vi "Spartan HTTP Load Global Resource Configuration.vi"(8 "error in (no error)":errorcluster) -> (0 "error out":errorcluster)   [LabVIEW 2011]
uses:
  ITK EXT/http/http0.llb/HTTP LVHTTP Global.vi
  ITK EXT/http/config.llb/HTTP SRM.vi
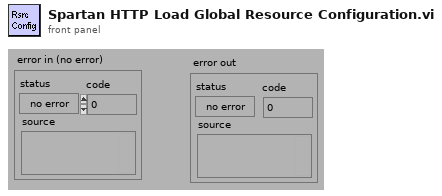
[diagram p1: front panel]
types:
  T1 = typedef "Keyed Array.ctl" = cluster{"keys":string[], "values":string[]}
  T2 = enum32{"noop", "DocumentRoot", "UserDir", "AccessFileName", "DefaultType", "DefaultIcon", "DirectoryIndex", "ReadmeName", "HeaderName", "ErrorDocument", "FancyIndexing", "IndexIgnore", "IndexOption", "Redirect", "Alias", "ScriptAlias", "AddType", "AddEncoding", "AddDescription", "AddIcon", "AddIconByType", "AddIconByEncoding"}
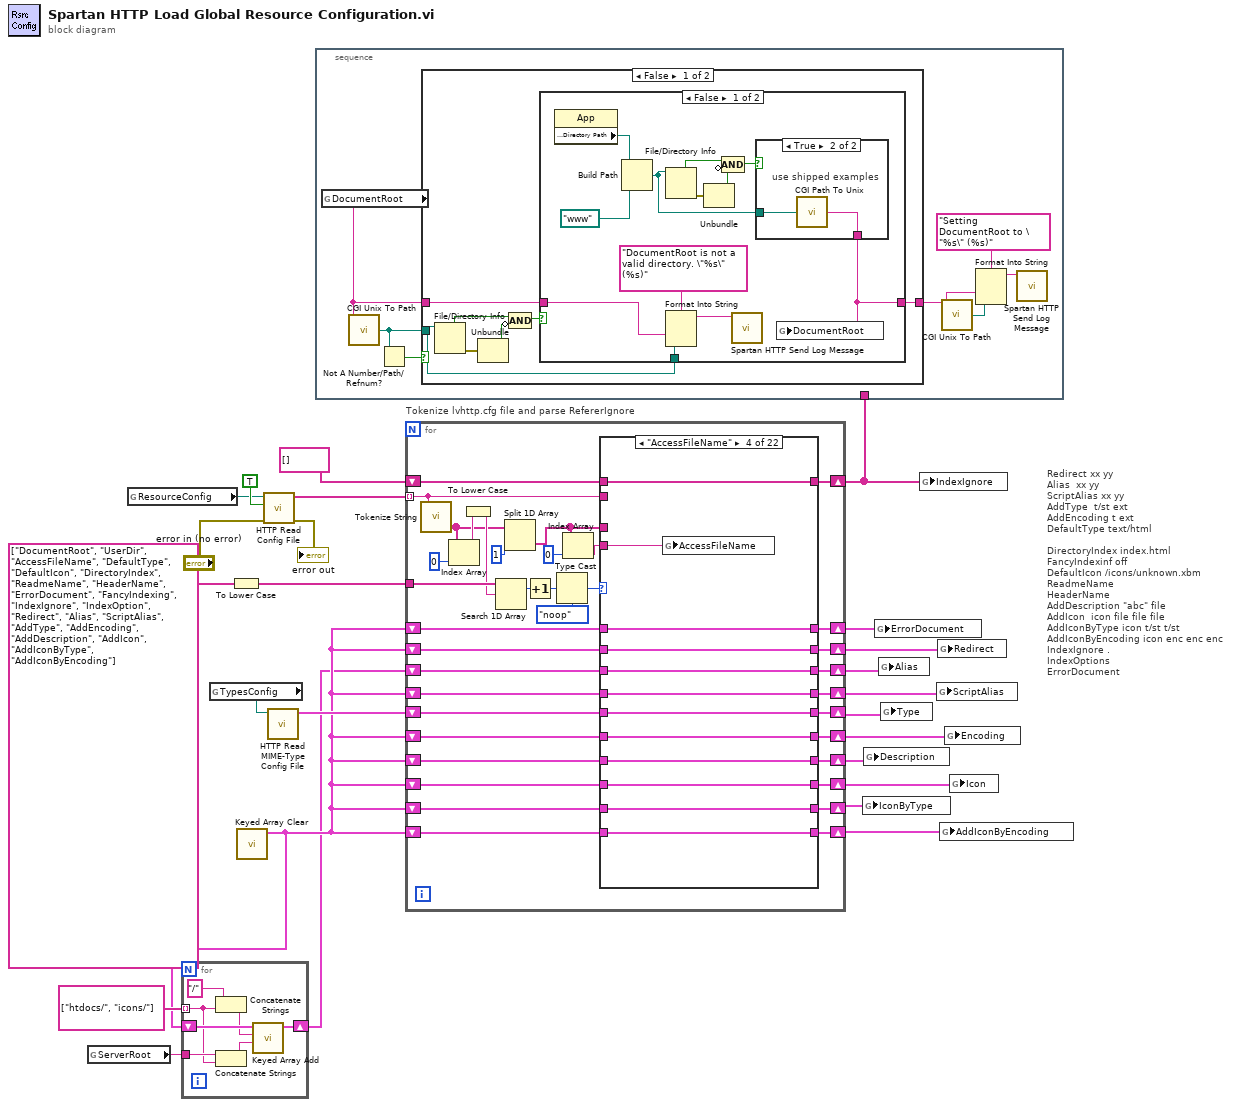
[diagram p0: block diagram]
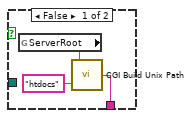
[diagram p2: hidden frame]
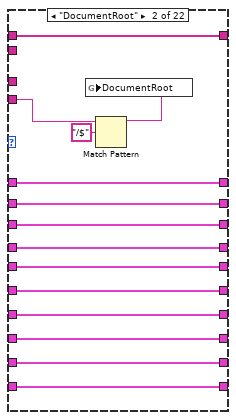
[diagram p6: hidden frame]
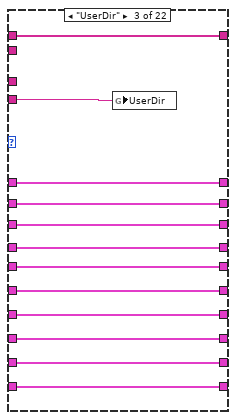
[diagram p7: hidden frame]
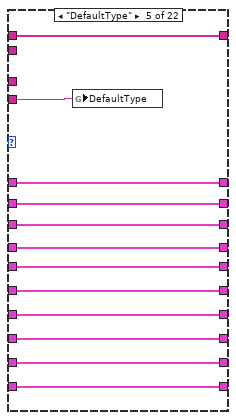
[diagram p8: hidden frame]
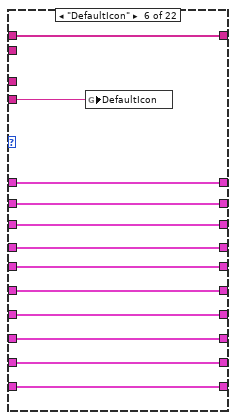
[diagram p9: hidden frame]
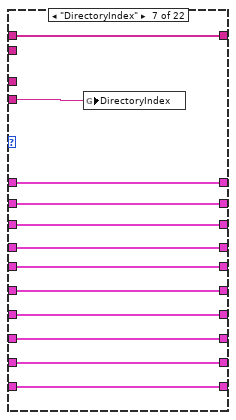
[diagram p10: hidden frame]
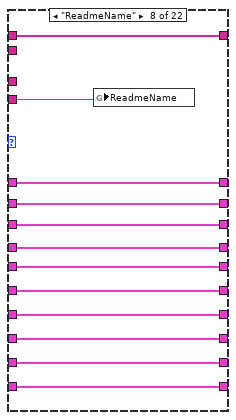
[diagram p11: hidden frame]
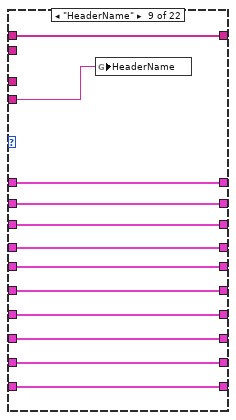
[diagram p12: hidden frame]
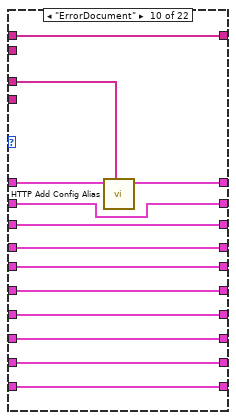
[diagram p13: hidden frame]
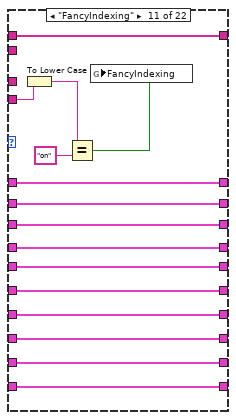
[diagram p14: hidden frame]
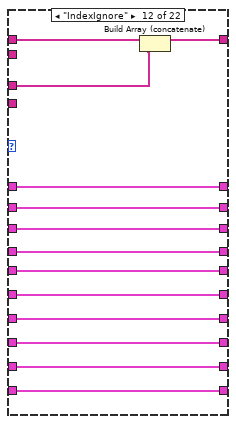
[diagram p15: hidden frame]
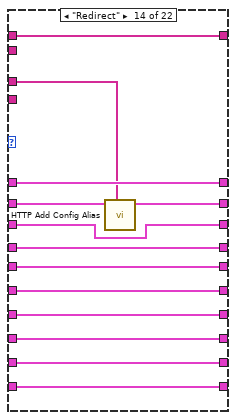
[diagram p17: hidden frame]
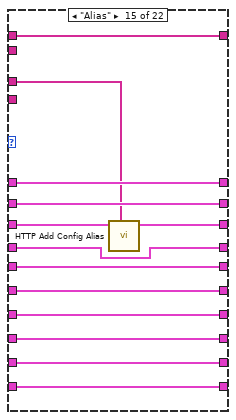
[diagram p18: hidden frame]
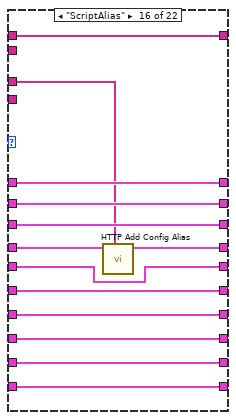
[diagram p19: hidden frame]
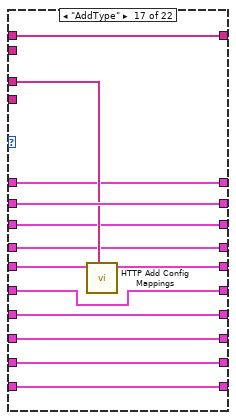
[diagram p20: hidden frame]
diagram:
  # "Redirect\txx yy\nAlias\t\txx yy\nScriptAlias\txx yy\nAddType\t\tt/st ext\nAddEncoding\tt ext\nDefaultType\ttext/html\n\nDirectoryIndex\tindex.html\nFancyIndexinf\toff\nDefaultIcon\t/icons/unknown.xbm\nReadmeName\nHeaderName\nAddDescription\t\"abc\" file\nAddIcon\t\ticon file file file\nAddIconByType\ticon t/st t/st\nAddIconByEncoding\ticon enc enc enc\nIndexIgnore\t.\nIndexOptions\nErrorDocument"
  n1 = global read "HTTP LVHTTP Global.vi" "ServerRoot"() -> (w14:string)
  n2 = global read "HTTP LVHTTP Global.vi" "ResourceConfig"() -> (w17:path)
  n3 = global read "HTTP LVHTTP Global.vi" "TypesConfig"() -> (w25:path)
  n4 = To Lower Case(string=string[] ["DocumentRoot", "UserDir", "AccessFileName", "DefaultType", "DefaultIcon", "DirectoryIndex", "ReadmeName", "HeaderName", "ErrorDocument", "FancyIndexing", "IndexIgnore", "IndexOption", "Redirect", "Alias", "ScriptAlias", "AddType", "AddEncoding", "AddDescription", "AddIcon", "AddIconByType", "AddIconByEncoding"] ("token array")) -> (all lower case string=w16:string[])
  n5 = call "Keyed Array Clear.vi"() -> ("array out"=w13:T1)  [unwired: 1 in, 6 out]
  n6 = for {
    shift-right: [w31] -> w12
    shift-left: w13 -> [w32]
    tunnel: string[] ["htdocs/", "icons/"] -> [w27] mode=indexing
    tunnel: w14 -> [w28]
    n7 = Concatenate Strings("/", w27) -> (w29:string)
    n8 = Concatenate Strings(w28, w27) -> (w26:string)
    n9 = call "Keyed Array Add.vi"("value"=w26, "key"=w29, "array in"=w32) -> ("array out"=w31:T1)  [unwired: 1 in, 3 out]
  }
  n10 = call "HTTP Read Config File.vi"("error in (no error)"="error in (no error)", "skip blank lines (F)"=TRUE, "config file path"=w17) -> ("error out"=→"error out":errorcluster, "lines"=w22:string[])  [unwired: 7 out]
  n11 = call "HTTP Read MIME-Type Config File.vi"("mime.types config file path"=w25) -> ("mime mapping"=w18:T1)  [unwired: 1 in, 9 out]
  n12 = for "Tokenize lvhttp.cfg file and parse RefererIgnore" {
    shift-right: [w47] -> w9
    shift-left: w13 -> [w68]
    tunnel: w22 -> [w40] mode=indexing
    shift-right: [w66] -> w11
    shift-left: string[] [] -> [w67]
    tunnel: w16 -> [w65]
    shift-right: [w60] -> w8
    shift-left: w12 -> [w61]
    shift-right: [w59] -> w7
    shift-left: w13 -> [w58]
    shift-right: [w56] -> w6
    shift-left: w18 -> [w57]
    shift-right: [w54] -> w5
    shift-left: w13 -> [w55]
    shift-right: [w53] -> w4
    shift-left: w13 -> [w46]
    shift-right: [w52] -> w3
    shift-left: w13 -> [w51]
    shift-right: [w50] -> w2
    shift-left: w13 -> [w49]
    shift-right: [w48] -> w1
    shift-left: w13 -> [w45]
    shift-right: [w44] -> w10
    shift-left: w13 -> [w43]
    n13 = call "Tokenize String.vi"("input string"=w40) -> ("token array"=w35:string[])  [unwired: 1 in, 3 out]
    n14 = Index Array(array=w35, index=0) -> (element=w38:string)
    n15 = To Lower Case(string=w38) -> (all lower case string=w42:string)
    n16 = Search 1D Array(1D array=w65, element=w42) -> (index of element=w41:i32)  [unwired: 1 out]
    n17 = Split 1D Array(array=w35, index=1) -> (second subarray=w34:string[])  [unwired: 1 out]
    n18 = Increment(x=w41) -> (x+1=w64:i32)
    n19 = Type Cast(type=T2."noop" ("ring copy"), x=w64) -> (*(type *) &x=w63:T2)
    n20 = Index Array(array=w34, index=0) -> (element=w36:string)
    n21 = case shown="\"AccessFileName\"" w63 {
      tunnel: w34 -> [_ _ _ _ _ _ _ _ _ w178 _ w206 _ w230 w243 w256 w278 w292 _ w318 w331 w344]
      tunnel: w67 -> [w79 w93 w96 w115 w120 w141 w153 w164 w177 w190 w204 w217 w229 w242 w255 w268 w281 w294 w307 w320 w333 w346]
      tunnel: [w79 w93 w96 w115 w120 w141 w153 w164 w177 w190 w204 w216 w229 w242 w255 w268 w281 w294 w307 w320 w333 w346] -> w66
      tunnel: w61 -> [w77 w91 w104 w116 w128 w139 w151 w163 w175 w182 w202 w215 w221 w233 w254 w259 w270 w283 w297 w309 w323 w335]
      tunnel: [w77 w91 w104 w116 w128 w139 w151 w163 w175 w182 w202 w215 w221 w233 w245 w259 w270 w283 w297 w309 w323 w335] -> w60
      tunnel: [w76 w90 w103 w114 w127 w138 w150 w162 w174 w183 w201 w214 w222 w234 w246 w258 w271 w284 w298 w310 w324 w336] -> w59
      tunnel: w58 -> [w76 w90 w103 w114 w127 w138 w150 w162 w174 w183 w201 w214 w222 w234 w246 w266 w271 w284 w298 w310 w324 w336]
      tunnel: w57 -> [w75 w89 w102 w113 w126 w137 w149 w161 w173 w179 w200 w213 w223 w235 w247 w260 w277 w285 w299 w311 w325 w337]
      tunnel: [w75 w89 w102 w113 w126 w137 w149 w161 w173 w179 w200 w213 w223 w235 w247 w260 w279 w285 w299 w311 w325 w337] -> w56
      tunnel: w55 -> [w74 w88 w101 w112 w125 w136 w148 w160 w172 w184 w199 w212 w224 w236 w248 w261 w272 w291 w300 w312 w326 w338]
      tunnel: [w74 w88 w101 w112 w125 w136 w148 w160 w172 w184 w199 w212 w224 w236 w248 w261 w272 w290 w300 w312 w326 w338] -> w54
      tunnel: [w73 w87 w100 w111 w124 w135 w147 w159 w171 w185 w198 w211 w225 w237 w249 w262 w273 w286 w304 w313 w327 w339] -> w53
      tunnel: [w72 w86 w99 w110 w123 w134 w146 w158 w170 w186 w197 w210 w226 w238 w250 w263 w274 w287 w301 w317 w328 w340] -> w52
      tunnel: w51 -> [w72 w86 w99 w110 w123 w134 w146 w158 w170 w186 w197 w210 w226 w238 w250 w263 w274 w287 w301 w316 w328 w340]
      tunnel: [w71 w85 w98 w109 w122 w133 w145 w157 w169 w187 w196 w209 w227 w239 w251 w264 w275 w288 w302 w314 w330 w341] -> w50
      tunnel: w49 -> [w71 w85 w98 w109 w122 w133 w145 w157 w169 w187 w196 w209 w227 w239 w251 w264 w275 w288 w302 w314 w329 w341]
      tunnel: [w70 w84 w97 w108 w121 w132 w144 w156 w168 w188 w195 w208 w228 w240 w252 w265 w276 w289 w303 w315 w322 w343] -> w48
      tunnel: w68 -> [w78 w92 w105 w117 w129 w140 w152 w165 w176 w189 w203 w218 w220 w241 w253 w267 w280 w293 w306 w319 w332 w345]
      tunnel: [w78 w92 w105 w117 w129 w140 w152 w165 w176 w189 w203 w218 w220 w232 w253 w267 w280 w293 w306 w319 w332 w345] -> w47
      tunnel: w46 -> [w73 w87 w100 w111 w124 w135 w147 w159 w171 w185 w198 w211 w225 w237 w249 w262 w273 w286 w305 w313 w327 w339]
      tunnel: w45 -> [w70 w84 w97 w108 w121 w132 w144 w156 w168 w188 w195 w208 w228 w240 w252 w265 w276 w289 w303 w315 w322 w342]
      tunnel: w40 -> [_ _ _ _ _ _ _ _ _ _ _ _ _ _ _ _ _ _ w296 _ _ _]
      tunnel: [w69 w83 w95 w107 w119 w131 w143 w155 w167 w180 w194 w207 w219 w231 w244 w257 w269 w282 w295 w308 w321 w334] -> w44
      tunnel: w43 -> [w69 w83 w95 w107 w119 w131 w143 w155 w167 w181 w194 w207 w219 w231 w244 w257 w269 w282 w295 w308 w321 w334]
      tunnel: w36 -> [_ w82 w94 w106 w118 w130 w142 w154 w166 _ w192 _ _ _ _ _ _ _ _ _ _ _]
      frame "noop" {
      }
      frame "DocumentRoot" {
        n22 = Match Pattern(string=w82, regular expression="/$") -> (before substring=w80:string)  [unwired: 4 out]
        n23 = global write "HTTP SRM.vi" "DocumentRoot"(w80) -> ()
      }
      frame "UserDir" {
        n24 = global write "HTTP SRM.vi" "UserDir"(w94) -> ()
      }
      frame "AccessFileName" {
        n25 = global write "HTTP SRM.vi" "AccessFileName"(w106) -> ()
      }
      frame "DefaultType" {
        n26 = global write "HTTP SRM.vi" "DefaultType"(w118) -> ()
      }
      frame "DefaultIcon" {
        n27 = global write "HTTP SRM.vi" "DefaultIcon"(w130) -> ()
      }
      frame "DirectoryIndex" {
        n28 = global write "HTTP SRM.vi" "DirectoryIndex"(w142) -> ()
      }
      frame "ReadmeName" {
        n29 = global write "HTTP SRM.vi" "ReadmeName"(w154) -> ()
      }
      frame "HeaderName" {
        n30 = global write "HTTP SRM.vi" "HeaderName"(w166) -> ()
      }
      frame "ErrorDocument" {
        n31 = call "HTTP Add Config Alias.vi"("token array"=w178, "array in"=w181) -> ("array out"=w180:T1)  [unwired: 9 out]
      }
      frame "FancyIndexing" {
        n32 = To Lower Case(string=w192) -> (all lower case string=w193:string)
        n33 = Equal?(x=w193, y="on") -> (x = y?=w191:bool)
        n34 = global write "HTTP SRM.vi" "FancyIndexing"(w191) -> ()
      }
      frame "IndexIgnore" {
        n35 = Build Array (concatenate)(w217, w206) -> (w216:string[])
      }
      frame "IndexOption" {
      }
      frame "Redirect" {
        n36 = call "HTTP Add Config Alias.vi"("token array"=w230, "array in"=w241) -> ("array out"=w232:T1)  [unwired: 9 out]
      }
      frame "Alias" {
        n37 = call "HTTP Add Config Alias.vi"("token array"=w243, "array in"=w254) -> ("array out"=w245:T1)  [unwired: 9 out]
      }
      frame "ScriptAlias" {
        n38 = call "HTTP Add Config Alias.vi"("token array"=w256, "array in"=w266) -> ("array out"=w258:T1)  [unwired: 9 out]
      }
      frame "AddType" {
        n39 = call "HTTP Add Config Mappings.vi"("token array"=w278, "array in"=w277) -> ("array out"=w279:T1)  [unwired: 1 in, 8 out]
      }
      frame "AddEncoding" {
        n40 = call "HTTP Add Config Mappings.vi"("token array"=w292, "array in"=w291) -> ("array out"=w290:T1)  [unwired: 1 in, 8 out]
      }
      frame "AddDescription" {
        n41 = call "HTTP Add Description Mapping.vi"("string"=w296, "array in"=w305) -> ("array out"=w304:T1)  [unwired: 9 out]
      }
      frame "AddIcon" {
        n42 = call "HTTP Add Config Icon Mappings.vi"("token array"=w318, "array in"=w316) -> ("array out"=w317:T1)  [unwired: 9 out]
      }
      frame "AddIconByType" {
        n43 = call "HTTP Add Config Icon Mappings.vi"("token array"=w331, "array in"=w329) -> ("array out"=w330:T1)  [unwired: 9 out]
      }
      frame "AddIconByEncoding" {
        n44 = call "HTTP Add Config Icon Mappings.vi"("token array"=w344, "array in"=w342) -> ("array out"=w343:T1)  [unwired: 9 out]
      }
    }
  }
  n45 = stacked-sequence {
    tunnel: w11 -> [_]
    frame #0 {
      n46 = global read "HTTP SRM.vi" "DocumentRoot"() -> (w347:string)
      n47 = call "CGI Unix To Path.vi"("unix path"=w347) -> ("platform path"=w350:path)  [unwired: 1 out]
      n48 = Not A Number/Path/Refnum?(number/path/refnum=w350) -> (NaN/Path/Refnum?=w351:bool)
      n49 = case shown="False" w351 {
        tunnel: w350 -> [w354 _]
        tunnel: w347 -> [w356 w379]
        tunnel: [w355 w379] -> w349
        frame False {
          n50 = File/Directory Info(path=w354) -> (directory=w358:bool, error out=w360:errorcluster)  [unwired: 1 in, 5 out]
          n51 = Unbundle(w360) -> ("status"=w359:bool)  [unwired: 2 out]
          n52 = Compound Arithmetic op=AND(w358, invert w359) -> (w357:bool)
          n53 = case shown="False" w357 {
            tunnel: w356 -> [w371 w378]
            tunnel: [w361 w378] -> w355
            tunnel: w354 -> [w370 _]
            frame False {
              n54 = property class="App"() -> ("Application:Directory Path"=w362:path)  [unwired: 2 in, 2 out]
              n55 = Build Path(base path=w362, name or relative path=path "www") -> (appended path=w363:path)
              n56 = File/Directory Info(path=w363) -> (directory=w367:bool, error out=w366:errorcluster)  [unwired: 1 in, 5 out]
              n57 = Format Into String(format string="DocumentRoot is not a valid directory. \"%s\" (%s)", w371, w370) -> (resulting string=w369:string)  [unwired: 2 in, 1 out]
              n58 = Unbundle(w366) -> ("status"=w368:bool)  [unwired: 2 out]
              n59 = Compound Arithmetic op=AND(w367, invert w368) -> (w364:bool)
              n60 = call "Spartan HTTP Send Log Message.vi"("message"=w369) -> ()  [unwired: 7 out]
              n61 = case shown="True" w364 {
                tunnel: [w373 w376] -> w361
                tunnel: w363 -> [_ w377]
                frame False {
                  n62 = global read "HTTP LVHTTP Global.vi" "ServerRoot"() -> (w375:string)
                  n63 = call "CGI Build Unix Path.vi"("absolute or relative path"="htdocs", "base path"=w375) -> ("new path"=w373:string)
                }
                frame True {
                  # "use shipped examples"
                  n64 = call "CGI Path To Unix.vi"("platform path"=w377) -> ("unix path"=w376:string)  [unwired: 1 in]
                }
              }
              n65 = global write "HTTP SRM.vi" "DocumentRoot"(w361) -> ()
            }
            frame True {
            }
          }
        }
        frame True {
        }
      }
      n66 = call "CGI Unix To Path.vi"("unix path"=w349) -> ("platform path"=w348:path)  [unwired: 1 out]
      n67 = Format Into String(format string="Setting DocumentRoot to \"%s\" (%s)", w349, w348) -> (resulting string=w352:string)  [unwired: 2 in, 1 out]
      n68 = call "Spartan HTTP Send Log Message.vi"("message"=w352) -> ()  [unwired: 7 out]
    }
  }
  n69 = global write "HTTP SRM.vi" "IconByType"(w2) -> ()
  n70 = global write "HTTP SRM.vi" "Description"(w4) -> ()
  n71 = global write "HTTP SRM.vi" "ErrorDocument"(w10) -> ()
  n72 = global write "HTTP SRM.vi" "Alias"(w8) -> ()
  n73 = global write "HTTP SRM.vi" "Type"(w6) -> ()
  n74 = global write "HTTP SRM.vi" "IndexIgnore"(w11) -> ()
  n75 = global write "HTTP SRM.vi" "ScriptAlias"(w7) -> ()
  n76 = global write "HTTP SRM.vi" "Redirect"(w9) -> ()
  n77 = global write "HTTP SRM.vi" "AddIconByEncoding"(w1) -> ()
  n78 = global write "HTTP SRM.vi" "Encoding"(w5) -> ()
  n79 = global write "HTTP SRM.vi" "Icon"(w3) -> ()
